vi "Draw.vi"(7 "Stimulus Snippet":T1, 8 "error in (no error)":errorcluster, 9 "StimulusImageIn":T2, 10 "CalibrationImage":T2, 11 "ConstantImageStimulus in":refnum<class "ConstantImageStimulus.lvclass">) -> (0 "error out":errorcluster, 1 "StimulusImageOut":T2, 3 "ConstantImageStimulus out":refnum<class "ConstantImageStimulus.lvclass">)   [LabVIEW 2019, in "ConstantImageStimulus.lvclass"]
uses:
  ConstantImageStimulus.lvclass
  <vilib>/vision/Image Controls.llb/IMAQ Image.ctl
  StimulusSnippetCluster.ctl
  ConstantImageStimulus.lvclass/ConstantImageStimulus.ctl
  ParametersGlobal.vi
  <vilib>/vision/NI_Vision_Development_Module.lvlib
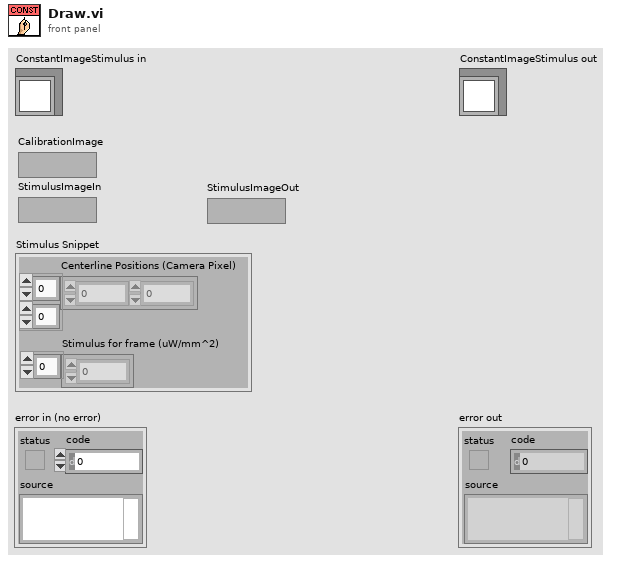
[diagram p1: front panel]
types:
  T1 = typedef "StimulusSnippetCluster.ctl" = cluster{"Centerline Positions (Camera Pixel)":sgl[][], "Stimulus for frame (uW/mm^2)":sgl[]}
  T2 = typedef "IMAQ Image.ctl" = refnum<image>
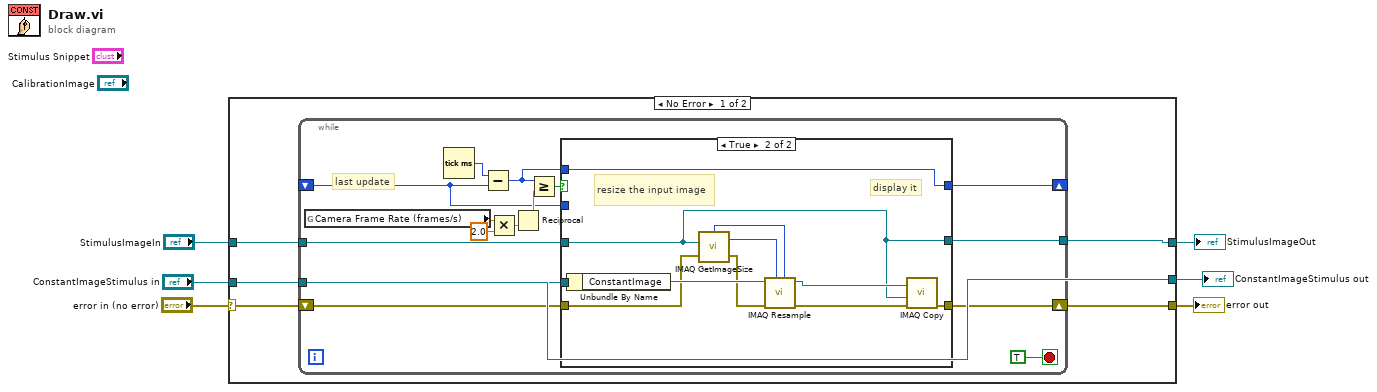
[diagram p0: block diagram]
diagram:
  n1 = case shown="No Error" "error in (no error)" {
    selector: "error in (no error)" -> [w11 w43]
    tunnel: "StimulusImageIn" -> [w8 w42]
    tunnel: [w9 w43] -> w4
    tunnel: [w7 w42] -> w3
    tunnel: "ConstantImageStimulus in" -> [w10 w41]
    tunnel: [w10 w41] -> w1
    frame No Error {
      n2 = while {
        tunnel: w10 -> [w25]
        tunnel: w8 -> [w23]
        shift-right: [w24] -> w9
        shift-left: w11 -> [w26]
        shift-right: [w18] -> _
        shift-left: _ -> [w16]
        tunnel: [w12] -> w7
        stop <- TRUE stop-if-true
        # "last update"
        n3 = global read "ParametersGlobal.vi" "Camera Frame Rate (frames/s)"() -> (w15:sgl)
        n4 = Tick Count (ms)() -> (millisecond timer value=w21:u32)
        n5 = Subtract(x=w21, y=w16) -> (x-y=w17:u32)
        n6 = Multiply(x=w15, y=sgl 2.0) -> (x*y=w14:sgl)
        n7 = Reciprocal(x=w14) -> (1/x=w20:sgl)
        n8 = Greater Or Equal?(x=w17, y=w20) -> (x >= y?=w19:bool)
        n9 = case shown="True" w19 {
          tunnel: w26 -> [w28 w39]
          tunnel: w25 -> [_ w38]
          tunnel: [w28 w36] -> w24
          tunnel: w23 -> [w27 w30]
          tunnel: [w29 w31] -> w18
          tunnel: w17 -> [_ w31]
          tunnel: w16 -> [w29 _]
          tunnel: [w27 w30] -> w12
          frame False {
            # "skip if we did this already this frame"
          }
          frame True {
            # "resize the input image"
            # "display it"
            n10 = Unbundle By Name(w38) -> ("ConstantImage"=w40:T2)
            n11 = call "IMAQ GetImageSize"("Image"=w30, "error in (no error)"=w39) -> ("Y Resolution"=w33:i32, "X Resolution"=w34:i32, "error out"=w32:errorcluster)  [unwired: 2 in]
            n12 = call "IMAQ Resample"("X Resolution"=w34, "Y Resolution"=w33, "error in (no error)"=w32, "Image Src"=w40) -> ("error out"=w37:errorcluster, "Image Dst Out"=w35:T2)  [unwired: 6 in]
            n13 = call "IMAQ Copy"("error in (no error)"=w37, "Image Dst"=w30, "Image Src"=w35) -> ("error out"=w36:errorcluster)  [unwired: 3 in, 1 out]
          }
        }
      }
    }
    frame Error {
    }
  }
  "error out" <- w4
  "ConstantImageStimulus out" <- w1
  "StimulusImageOut" <- w3
